vi "Read Greater_.vi"(8 "error in (no error)":errorcluster, 11 "AssertCompareValue in":refnum<class "AssertCompareValue.lvclass">) -> (0 "error out":errorcluster, 2 "Greater?":bool, 3 "AssertCompareValue out":refnum<class "AssertCompareValue.lvclass">)   [LabVIEW 2021, in "Bananas.lvlib" / "AssertCompareValue.lvclass"]
uses:
  AssertCompareValue.lvclass
  AssertCompareValue.lvclass/AssertCompareValue.ctl
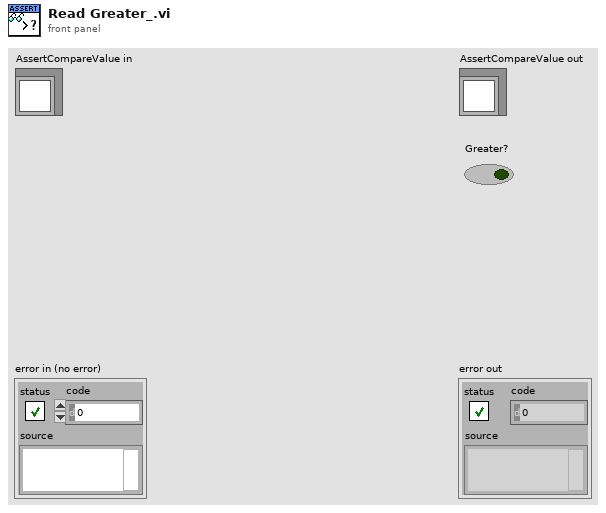
[diagram p1: front panel]
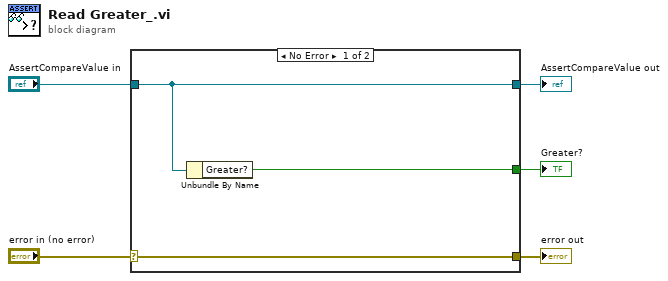
[diagram p0: block diagram]
diagram:
  n1 = case shown="No Error" "error in (no error)" {
    selector: "error in (no error)" -> [w8 w9]
    tunnel: [w8 w9] -> w4
    tunnel: [w7 w10] -> w2
    tunnel: "AssertCompareValue in" -> [w7 w10]
    tunnel: [w6 _] -> w1
    frame No Error {
      n2 = Unbundle By Name(w7) -> ("Greater?"=w6:bool)
    }
    frame Error {
    }
  }
  "error out" <- w4
  "AssertCompareValue out" <- w2
  "Greater?" <- w1
